vi "My_Control.vi"() -> ()   [LabVIEW 2024]
uses:
  <vilib>/DAQmx/read.llb/DAQmx Read (Analog 1D Wfm NChan NSamp).vi
  <vilib>/DAQmx/create/channels.llb/DAQmx Create Channel (AI-Voltage-Basic).vi
  <vilib>/DAQmx/configure/timing.llb/DAQmx Timing (Sample Clock).vi
  <vilib>/DAQmx/miscellaneous.llb/DAQmx Fill In Error Info.vi
  <vilib>/Waveform/WDTOps.llb/WDT Index Channel DBL.vi
  <vilib>/Analysis/2dsp.llb/Decimate (continuous, DBL).vi
  <vilib>/Analysis/NI_AALPro.lvlib
panel:
  in  "Tamaño ventana WL":i32=60
  in  "WL":dbl
  out "Waveform length":dbl[][](graph)
  out "number":u32
  in  "Limite superior WL":dbl=50.0
  in  "Limite inferior WL":dbl=25.0 format="%#_13g"
  in  "Escala autom. Y":u8=1
  in  "Maximo escala Y":dbl format="%#_13g"
  in  "Minimo escala Y":dbl format="%#_13g"
  in  "Minimo escala X":dbl
  in  "Maximo escala X":dbl
  in  "Escala autom. X":u8=1
  in  "Parar adquisicion 2":bool
  in  "factor decimacion":i32=20
  in  "tamaño buffer":i32=1000
  in  "Frecuencia muestreo":i32=20000
  in  "DAQmx Physical Channel":tag
  out "Senal EMG":waveform(dbl)[](graph)
  in  "Parar adquisicion":bool
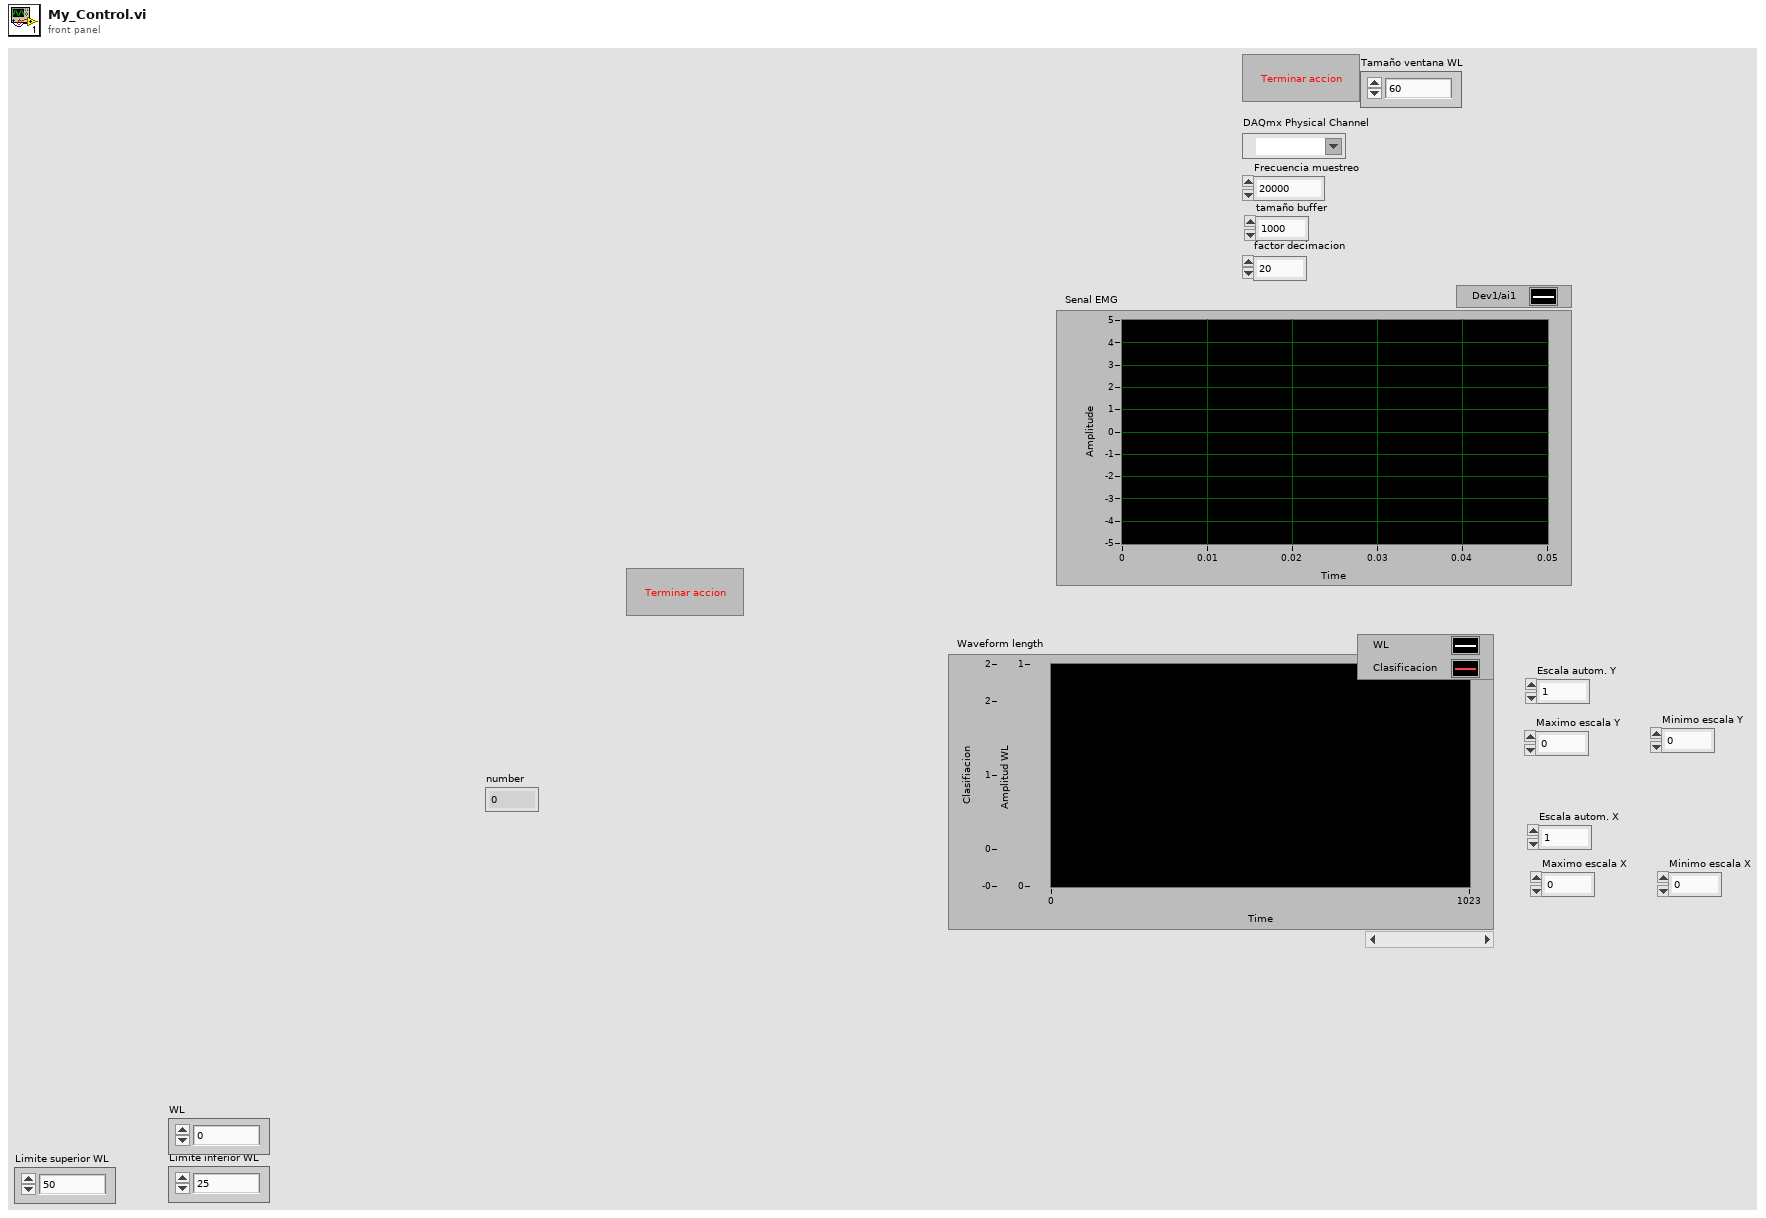
[diagram p1: front panel]
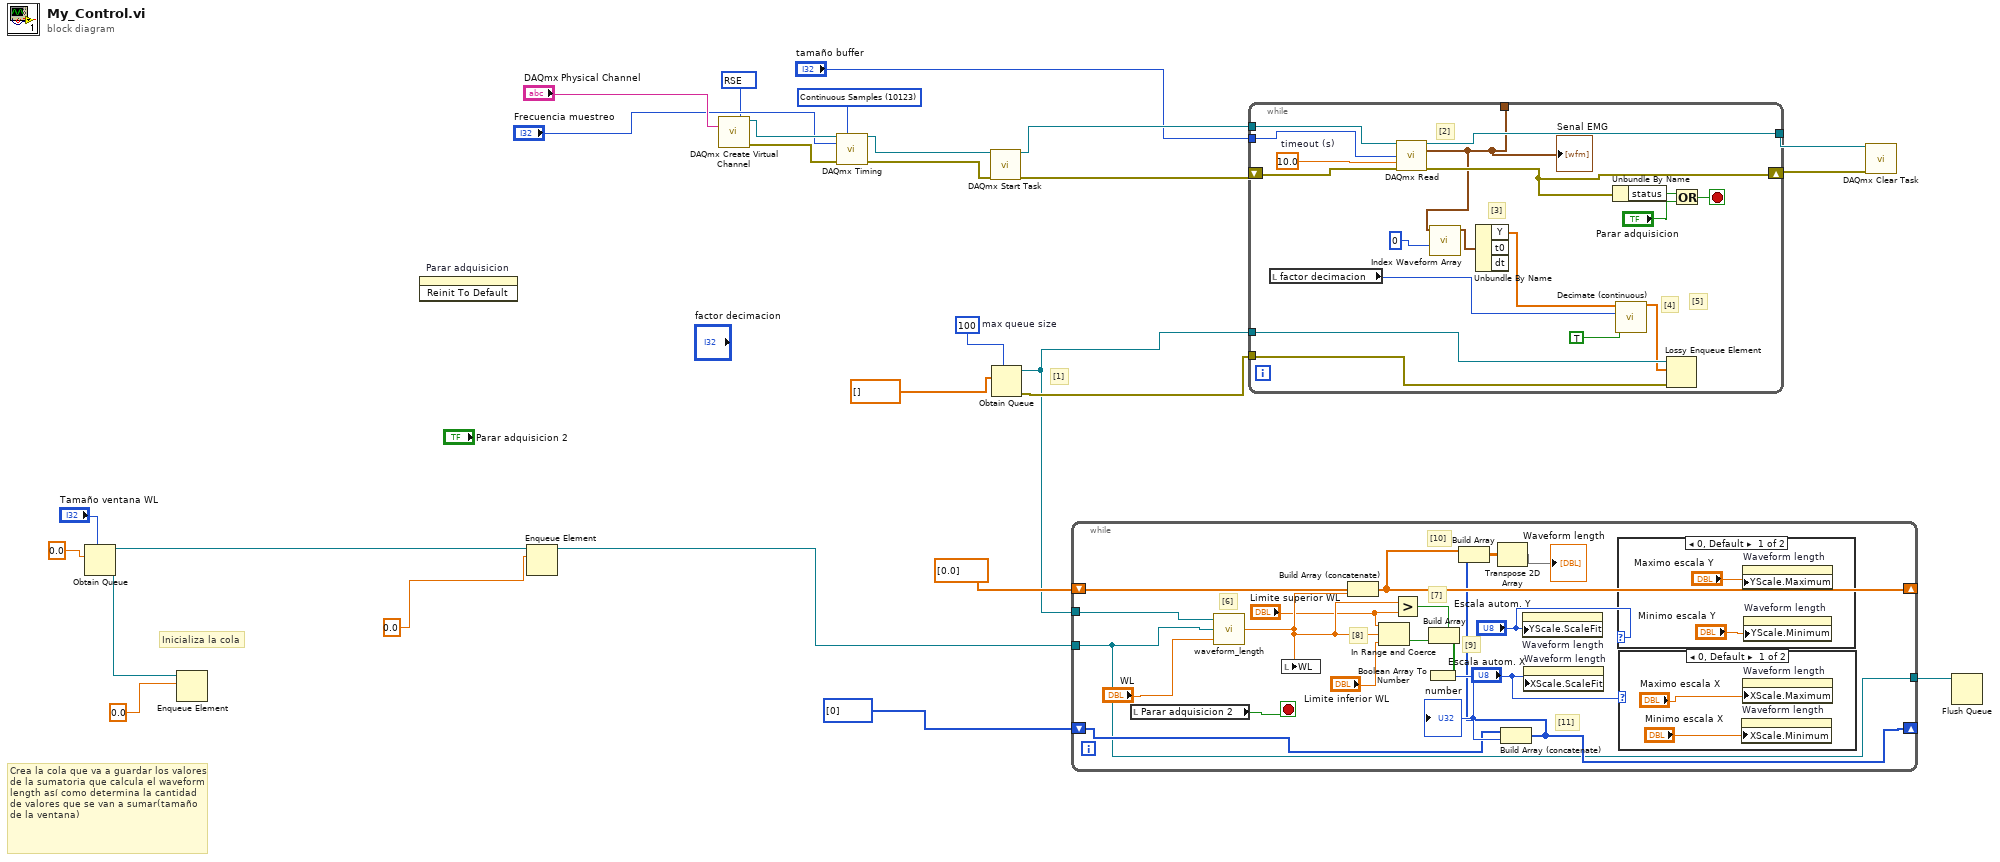
[diagram p0: block diagram]
diagram:
  w11 = 10123 items=["Finite Samples"=10178, "Continuous Samples"=10123, "Hardware Timed Single Point"=12522] ("sample mode")
  w12 = 10083 items=["Default"=-1, "RSE"=10083, "NRSE"=10078, "Differential"=10106, "Pseudodifferential"=12529] ("input terminal configuration")
  w21 = 100  # max queue size
  # "Inicializa la cola"
  # "Crea la cola que va a guardar los valores de la sumatoria que calcula el waveform length así como determina la cantidad de valores que se van a sumar(tamaño de la ventana)"
  # "[1]"
  n1 = Obtain Queue(max queue size (-1, unlimited)="Tamaño ventana WL", element data type=0.0) -> (queue out=w1:refnum<queue>)  [unwired: 3 in, 2 out]
  n2 = Enqueue Element(queue=w1, element=0.0) -> ()  [unwired: 2 in, 3 out]
  n3 = invoke on="Parar adquisicion" class="Bool (strict)" method="Reinit To Default"() -> ()  [unwired: 3 in, 3 out]
  n4 = Enqueue Element(queue=w1, element=0.0) -> (queue out=w8:refnum<queue>)  [unwired: 2 in, 2 out]
  n5 = call-poly <vilib>:"DAQmx Create Virtual Channel.vi"("input terminal configuration"=w12, "physical channels"="DAQmx Physical Channel") -> ("task out"=w18:refnum<k21>, "error out"=w17:errorcluster)  [unwired: 12 in]
  n6 = call-poly <vilib>:"DAQmx Timing.vi"("task/channels in"=w18, "sample mode"=w11, "rate"="Frecuencia muestreo", "error in"=w17) -> ("task out"=w16:refnum<k21>, "error out"=w15:errorcluster)  [unwired: 10 in]
  n7 = call <vilib>:"DAQmx Start Task.vi"("task/channels in"=w16, "error in"=w15) -> ("task out"=w26:refnum<k21>, "error out"=w25:errorcluster)  [unwired: 12 in]
  n8 = Obtain Queue(max queue size (-1, unlimited)=w21, element data type=dbl[] [] ("Cola tipo")) -> (queue out=w2:refnum<queue>, error out=w19:errorcluster)  [unwired: 3 in, 1 out]
  n9 = while {
    tunnel: w8 -> [w28]
    tunnel: w2 -> [w45]
    shift-right: [w31] -> _
    shift-left: dbl[] [0.0] -> [w42]
    shift-right: [w30] -> _
    shift-left: u32[] [0] -> [w32]
    tunnel: [w28] -> w6
    stop <- w43 stop-if-true
    # "[11]"
    # "[10]"
    # "[9]"
    # "[8]"
    # "[7]"
    # "[6]"
    n10 = local read "Parar adquisicion 2"() -> (w43:bool)
    n11 = call "waveform_length.vi"("WL"="WL", "Cola WL"=w28, "Datos entrada"=w45) -> ("WL 2"=w40:dbl)
    n12 = local write "WL"(w40) -> ()
    n13 = Build Array (concatenate)(w42, w40) -> (w31:dbl[])
    n14 = In Range and Coerce(upper limit="Limite superior WL", x=w40, lower limit="Limite inferior WL") -> (In Range?=w38:bool)  [unwired: 1 out]
    n15 = Greater?(x=w40, y="Limite superior WL") -> (0:w39:bool)
    n16 = Build Array(w39, w38) -> (w37:bool[])
    n17 = Boolean Array To Number(Boolean array=w37) -> (number=w33:u32)
    "number" <- w33
    n18 = Build Array (concatenate)(w32, w33) -> (w30:u32[])
    n19 = Build Array(w31, w30) -> (w29:dbl[][])
    n20 = Transpose 2D Array(2D array=w29) -> (transposed array=→"Waveform length":dbl[][])
    n21 = property on="Waveform length" class="WFChart (strict)"("YScale.ScaleFit"="Escala autom. Y") -> ()  [unwired: 2 in, 2 out]
    n22 = property on="Waveform length" class="WFChart (strict)"("XScale.ScaleFit"="Escala autom. X") -> ()  [unwired: 2 in, 2 out]
    n23 = case shown="0, Default" "Escala autom. Y" {
      frame 0, Default {
        n24 = property on="Waveform length" class="WFChart (strict)"("YScale.Maximum"="Maximo escala Y") -> ()  [unwired: 2 in, 2 out]
        n25 = property on="Waveform length" class="WFChart (strict)"("YScale.Minimum"="Minimo escala Y") -> ()  [unwired: 2 in, 2 out]
      }
      frame 1 {
      }
    }
    n26 = case shown="0, Default" "Escala autom. X" {
      frame 0, Default {
        n27 = property on="Waveform length" class="WFChart (strict)"("XScale.Minimum"="Minimo escala X") -> ()  [unwired: 2 in, 2 out]
        n28 = property on="Waveform length" class="WFChart (strict)"("XScale.Maximum"="Maximo escala X") -> ()  [unwired: 2 in, 2 out]
      }
      frame 1 {
      }
    }
  }
  n29 = while {
    tunnel: w26 -> [w67]
    tunnel: "tamaño buffer" -> [w64]
    tunnel: [w65] -> w22
    shift-right: [w62] -> w23
    shift-left: w25 -> [w66]
    tunnel: [w56] -> _
    tunnel: w2 -> [w52]
    tunnel: w19 -> [w51]
    stop <- w61 stop-if-true
    w60 = 10.0  # timeout (s)
    # "[5]"
    # "[4]"
    # "[3]"
    # "[2]"
    n30 = local read "factor decimacion"() -> (w53:i32)
    n31 = call-poly <vilib>:"DAQmx Read.vi"("task/channels in"=w67, "number of samples per channel"=w64, "timeout"=w60, "error in"=w66) -> ("task out"=w65:refnum<k21>, "data"=w56:waveform(dbl)[], "error out"=w62:errorcluster)  [unwired: 9 in]
    "Senal EMG" <- w56
    n32 = call-poly <vilib>:"Index Waveform Array.vi"("index"=0, "waveform array"=w56) -> ("waveform"=w57:waveform(dbl))  [unwired: 8 in, 1 out]
    n33 = Unbundle By Name(w57) -> ("Y"=w54:dbl[])  [unwired: 2 out]
    n34 = Unbundle By Name(w62) -> ("status"=w63:bool)
    n35 = call-poly <vilib>:"Decimate (continuous).vi"("averaging"=TRUE, "decimating factor"=w53, "X"=w54) -> ("Decimated Array"=w50:dbl[])  [unwired: 7 in, 1 out]
    n36 = Lossy Enqueue Element(queue=w52, element=w50, error in (no error)=w51) -> ()  [unwired: 4 out]
    n37 = Or(x=w63, y="Parar adquisicion") -> (x .or. y?=w61:bool)
  }
  n38 = call <vilib>:"DAQmx Clear Task.vi"("task in"=w22, "error in"=w23) -> ()  [unwired: 13 in, 1 out]
  n39 = Flush Queue(queue=w6) -> ()  [unwired: 1 in, 3 out]
